vi "Waveform Outputs.vi"(8 "error in (no error)":errorcluster, 11 "Node Ptr":T1 format="%.0x") -> (0 "error out":errorcluster)   [LabVIEW 2016, in "FPGA Addon System Explorer.lvlib"]
uses:
  FPGA Addon System Explorer.lvlib
  <vilib>/NI Veristand/Custom Device API/Custom Device Item Ref.ctl
  SubVIs/Channel Type.ctl
  Shared/get fpga resource values for cd group.vi
  FPGA-Resource-Manager-APIs/Source/find Relative VS Ref.vi
  FPGA-Resource-Manager-APIs/Source/get fgpa resources.vi
  <vilib>/NI VeriStand/Custom Device API/Custom Device API.lvlib
  FPGA-Resource-Manager-APIs/Source/FPGA RM Client API.lvlib
panel:
  in  "remove":bool
  in  "add":bool
  in  "Available DMA":i32[](listbox)
  in  "Header 2":cluster{"Section Name":string}={"Section Name"="Custom Device Item Settings"}
  in  "SHDocVw.IWebBrowser":refnum<k7>(container)
  in  "Header":cluster{"Section Name":string}={"Section Name"="Custom Device Item Settings"}
  in  "Description":string
  out "Name":string
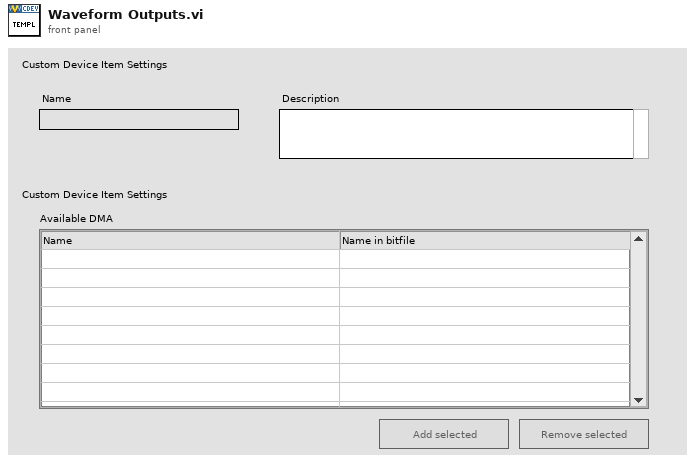
[diagram p1: front panel]
types:
  T1 = typedef "Custom Device API.lvlib/Custom Device Item Ref.ctl" = u64
  T2 = typedef "Custom Device API.lvlib/Custom Device Item Info.ctl" = cluster{"Name":string, "Is Channel":bool, "GUID":string, "Is Waveform":bool}
  T3 = typedef "Fifo_DMA_Config.ctl" = cluster{"Name":string, "Depth":u32, "Write? (Deprecated:Use Implementation)":bool, "Physical Channel":u32, "Base Address":u32, "Data Width":u32, "Data Type":T4, "FXP Properties":variant, "Write Window Address":u32, "Implementation":T5, "Control Set":u32}
  T4 = typedef "niFpgaDataTypeControl.ctl" = enum32{"Boolean", "I8", "I16", "I32", "I64", "U8", "U16", "U32", "U64", "FXP", "CustomControl", "SGL"}
  T5 = typedef "niFpgaDmaChannelImplementation.ctl" = enum16{"niFpgaTargetToHost", "niFpgaHostToTarget", "niFpgaPeerToPeerWriter", "niFpgaPeerToPeerReader", "niCoreTargetToHost", "niCoreHostToTarget"}
  T6 = typedef "FPGA Addon System Explorer.lvlib/Listbox Cluster.ctl" = cluster{"add":refnum<vi>, "remove":refnum<vi>, "Listbox":refnum<vi>, "selected":i32[], "not present":i32[], "reserved":i32[], "listbox text":string[][], "Section Ref":T1}
  T7 = typedef "FPGA RM Client API.lvlib/Channel Type.ctl" = enum16{"Write Channel", "Read Channel", "Write Waveform", "Read Waveform"}
  T8 = typedef "Custom Device API.lvlib/Custom Device Commands.ctl" = enum16{"Default", "Item renamed", "Shutdown", "Dynamic button pressed"}
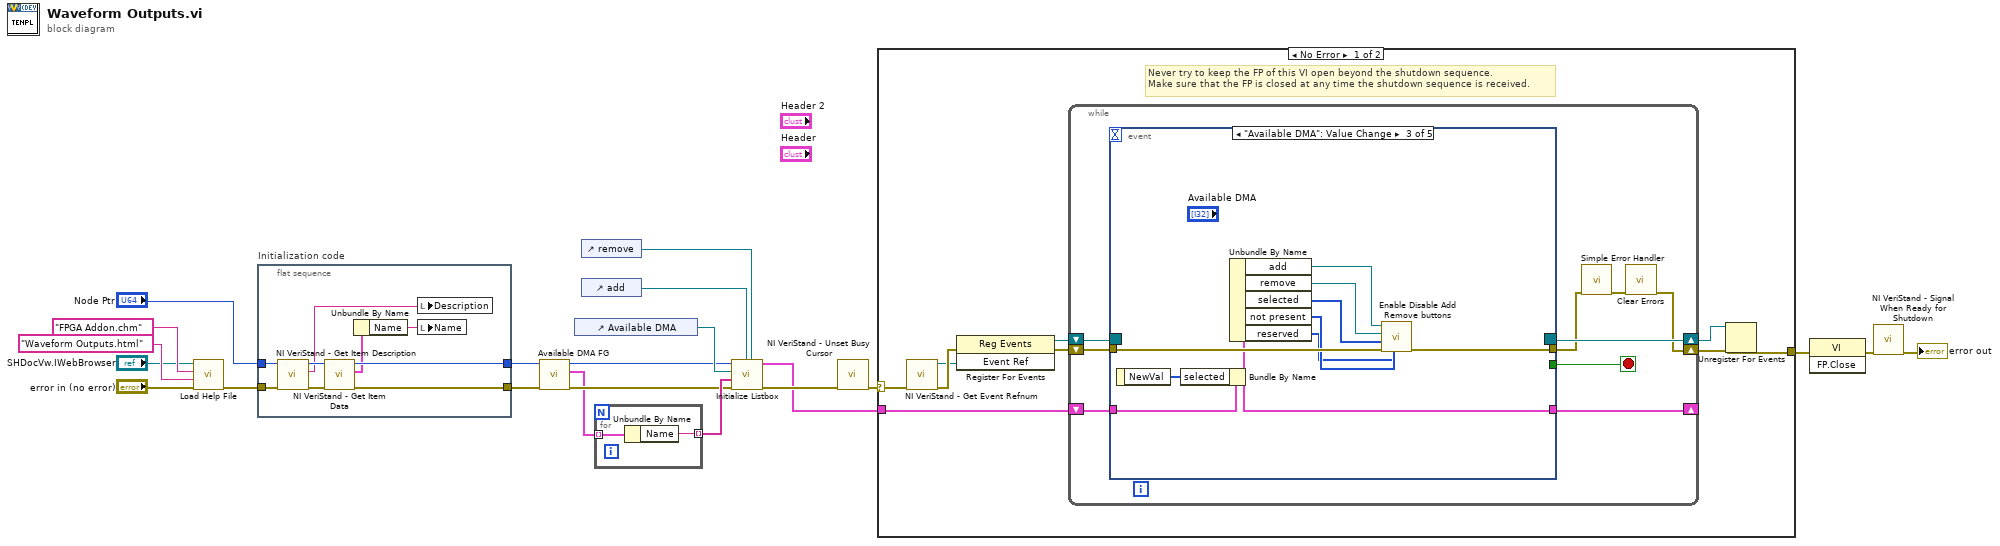
[diagram p0: block diagram]
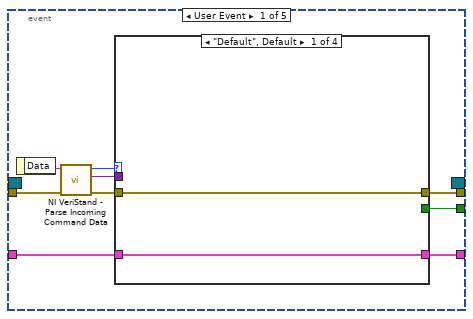
[diagram p2: hidden frame]
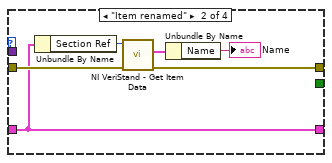
[diagram p3: hidden frame]
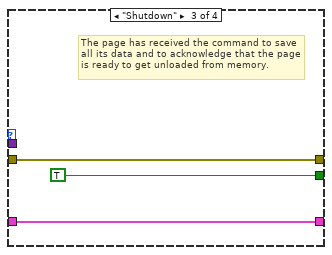
[diagram p4: hidden frame]
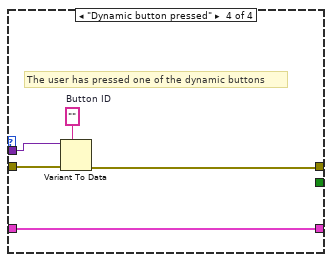
[diagram p5: hidden frame]
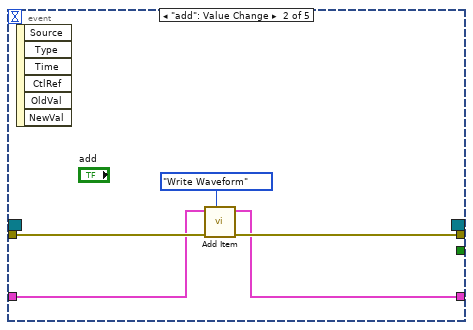
[diagram p6: hidden frame]
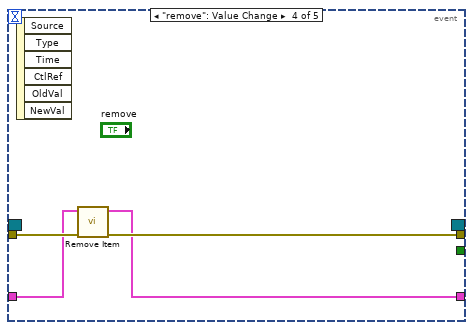
[diagram p7: hidden frame]
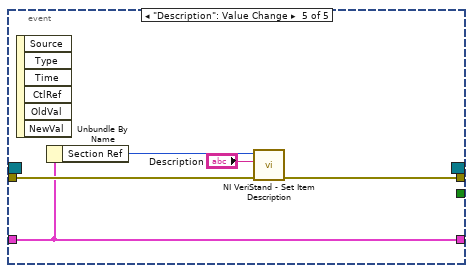
[diagram p8: hidden frame]
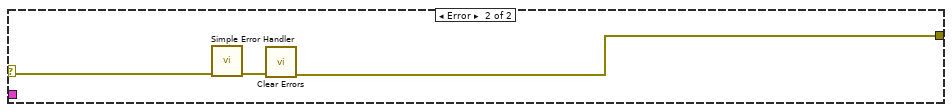
[diagram p9: hidden frame]
diagram:
  n1 = call "Load Help File.vi"("error in (no error)"="error in (no error)", "HTML File"="Waveform Outputs.html", "Main CHM File"="FPGA Addon.chm", "SHDocVw.IWebBrowser2"="SHDocVw.IWebBrowser") -> ("error out"=w16:errorcluster)  [unwired: 7 in]
  n2 = flat-sequence "Initialization code" {
    tunnel: w16 -> [w28]
    tunnel: "Node Ptr" -> [w27]
    tunnel: [w22] -> w5
    tunnel: [w30] -> w4
    frame #0 {
      n3 = call <vilib>:"NI VeriStand - Get Item Description.vi"("error in (no error)"=w28, "Item Ref in"=w27) -> ("error out"=w25:errorcluster, "Description"=w26:string, "Item Ref out"=w29:T1)  [unwired: 7 out]
      n4 = call <vilib>:"NI VeriStand - Get Item Data.vi"("error in (no error)"=w25, "Item Ref in"=w29) -> ("error out"=w22:errorcluster, "Item Info"=w24:T2, "Item Ref out"=w30:T1)  [unwired: 7 out]
      n5 = Unbundle By Name(w24) -> ("Name"=w23:string)
      n6 = local write "Description"(w26) -> ()
      n7 = local write "Name"(w23) -> ()
    }
  }
  n8 = call "Available DMA FG.vi"("error in (no error)"=w5, "Item Ref"=w4) -> ("error out"=w3:errorcluster, "Available DMA"=w2:T3[], "Item Ref out"=w1:T1)  [unwired: 7 in]
  n9 = control-ref of="Available DMA"() -> (w10:refnum<vi>)
  n10 = control-ref of="remove"() -> (w13:refnum<vi>)
  n11 = control-ref of="add"() -> (w14:refnum<vi>)
  n12 = for {
    tunnel: w2 -> [w32] mode=indexing
    tunnel: [w31] -> w15 mode=indexing
    n13 = Unbundle By Name(w32) -> ("Name"=w31:string)
  }
  n14 = call "Initialize Listbox.vi"("remove"=w13, "add"=w14, "error in (no error)"=w3, "Names"=w15, "Listbox"=w10, "Item Ref"=w1) -> ("error out"=w12:errorcluster, "Listbox Refs"=w11:T6)  [unwired: 4 in]
  n15 = call <vilib>:"NI VeriStand - Unset Busy Cursor.vi"("error in (no error)"=w12) -> ("error out"=w19:errorcluster)  [unwired: 10 out]
  n16 = case shown="No Error" w19 {
    selector: w19 -> [w34 w102]
    tunnel: [w38 w100] -> w21
    tunnel: w11 -> [w33 _]
    frame No Error {
      # "Never try to keep the FP of this VI open beyond the shutdown sequence.\nMake sure that the FP is closed at any time the shutdown sequence is received."
      n17 = call <vilib>:"NI VeriStand - Get Event Refnum.vi"("error in (no error)"=w34) -> ("error out"=w41:errorcluster, "Event Ref"=w37:refnum<user-event>)  [unwired: 9 out]
      n18 = register-events(error in=w41, w37) -> (reference out=w35:refnum<event-registration>, error out=w36:errorcluster)  [unwired: 1 in]
      n19 = while {
        shift-right: [w44] -> w39
        shift-left: w36 -> [w49]
        shift-right: [w50] -> w40
        shift-left: w35 -> [w48]
        shift-right: [w42] -> _
        shift-left: w33 -> [w43]
        stop <- w47 stop-if-true
        n20 = event shown="[2] \"Available DMA\": Value Change" {
          selector: w48 -> [_ _ _ _ _]
          dyn-events: [_ _ _ _ _] -> w50
          timeout: _ -> [_ _ _ _ _]
          tunnel: w49 -> [w59 w80 w90 w93 w99]
          tunnel: [w55 _ _ _ _] -> w47
          tunnel: [w54 w79 w89 w94 w98] -> w46
          tunnel: w43 -> [w52 w77 w87 w92 w97]
          tunnel: [w51 w78 w86 w91 w97] -> w42
          event User Event {
            n21 = event-data() -> ("Data"=w58:string)  [unwired: 1 out]
            n22 = call <vilib>:"NI VeriStand - Parse Incoming Command Data.vi"("error in (no error)"=w59, "Incoming data"=w58) -> ("error out"=w57:errorcluster, "Outgoing data"=w53:variant, "Action"=w56:T8)  [unwired: 7 out]
            n23 = case shown="\"Default\", Default" w56 {
              tunnel: w57 -> [w61 w67 w69 w75]
              tunnel: [_ _ TRUE _] -> w55
              tunnel: [w61 w65 w69 w72] -> w54
              tunnel: w53 -> [_ _ _ w74]
              tunnel: w52 -> [w60 w63 w68 w71]
              tunnel: [w60 w63 w68 w71] -> w51
              frame "Default", Default {
              }
              frame "Item renamed" {
                n24 = Unbundle By Name(w63) -> ("Section Ref"=w64:T1)
                n25 = call <vilib>:"NI VeriStand - Get Item Data.vi"("error in (no error)"=w67, "Item Ref in"=w64) -> ("error out"=w65:errorcluster, "Item Info"=w66:T2)  [unwired: 8 out]
                n26 = Unbundle By Name(w66) -> ("Name"=→"Name":string)
              }
              frame "Shutdown" {
                # "The page has received the command to save all its data and to acknowledge that the page is ready to get unloaded from memory."
              }
              frame "Dynamic button pressed" {
                w73 = ""  # Button ID
                # "The user has pressed one of the dynamic buttons"
                n27 = Variant To Data(error in=w75, type=w73, Variant=w74) -> (error out=w72:errorcluster)  [unwired: 1 out]
              }
            }
          }
          event "add": Value Change {
            n28 = event-data() -> ()  [unwired: 7 out]
            n29 = call "Add Item.vi"("Action"=Channel_Type."Write Waveform", "error in (no error)"=w80, "Listbox Refs in"=w77) -> ("error out"=w79:errorcluster, "Listbox Refs out"=w78:T6)  [unwired: 7 in]
          }
          event "Available DMA": Value Change {
            n30 = event-data() -> ("NewVal"=w85:i32[])  [unwired: 1 out]
            n31 = Bundle By Name(cluster=w87, "selected"=w85) -> (w86:T6)
            n32 = Unbundle By Name(w86) -> ("add"=w82:refnum<vi>, "remove"=w83:refnum<vi>, "selected"=w84:i32[], "not present"=w88:i32[], "reserved"=w81:i32[])
            n33 = call "Enable Disable Add Remove buttons.vi"("reserved item indexes"=w81, "not present item indexes"=w88, "error in (no error)"=w90, "selected items"=w84, "remove button"=w83, "add button"=w82) -> ("error out"=w89:errorcluster)  [unwired: 5 in]
          }
          event "remove": Value Change {
            n34 = event-data() -> ()  [unwired: 7 out]
            n35 = call "Remove Item.vi"("error in (no error)"=w93, "Listbox Refs in"=w92) -> ("error out"=w94:errorcluster, "Listbox Refs out"=w91:T6)  [unwired: 8 in]
          }
          event "Description": Value Change {
            n36 = event-data() -> ()  [unwired: 7 out]
            n37 = Unbundle By Name(w97) -> ("Section Ref"=w96:T1)
            n38 = call <vilib>:"NI VeriStand - Set Item Description.vi"("error in (no error)"=w99, "Description"="Description", "Item Ref in"=w96) -> ("error out"=w98:errorcluster)  [unwired: 8 out]
          }
        }
        n39 = call <vilib>:"Simple Error Handler.vi"("error in (no error)"=w46) -> ("error out"=w45:errorcluster)  [unwired: 1 in, 7 out]
        n40 = call <vilib>:"Clear Errors.vi"("error in (no error)"=w45) -> ("error out"=w44:errorcluster)  [unwired: 1 in, 5 out]
      }
      n41 = Unregister For Events(event registration refnum=w40, error in=w39) -> (error out=w38:errorcluster)
    }
    frame Error {
      n42 = call <vilib>:"Simple Error Handler.vi"("error in (no error)"=w102) -> ("error out"=w101:errorcluster)  [unwired: 1 in, 7 out]
      n43 = call <vilib>:"Clear Errors.vi"("error in (no error)"=w101) -> ("error out"=w100:errorcluster)  [unwired: 1 in, 5 out]
    }
  }
  n44 = invoke class="VI" method="FP.Close"(error in=w21) -> (error out=w20:errorcluster)  [unwired: 2 in, 2 out]
  n45 = call <vilib>:"NI VeriStand - Signal When Ready for Shutdown.vi"("error in (no error)"=w20) -> ("error out"=→"error out":errorcluster)  [unwired: 10 out]
